vi "Tell Self Forward.vi"(6 "Msg":refnum<class "Msg.lvclass">, 7 "Actor in":refnum<class "Actor.lvclass">, 9 "Msg Attributes":T1 {"Teller"."Absolute Time" format="%<%x %.3X>T"}, 10 "Previous Told":bool) -> (0 "Error out":errorcluster, 1 "Told":bool, 2 "Told Or Previous Told":bool, 5 "Actor out":refnum<class "Actor.lvclass">)   [LabVIEW 2020, in "_Template.lvlib" / "Templates.lvlib" / "TEMPLATE jettl Msg.lvlib" / "TEMPLATE.lvlib"]
uses:
  TEMPLATE/TEMPLATE.lvlib
  jettl/jettl/jettl.lvlib
  jettl/jettl/Actor/Actor.lvclass
  jettl/jettl/Msg Input/Msg Input.lvclass
  jettl/jettl/Msg Output/Msg Output.lvclass
  jettl/jettl/Msg/Msg.lvclass
  jettl/jettl/Relation.ctl
  jettl/jettl/Teller.ctl
  jettl/jettl/Msg Attributes.ctl
panel:
  # "This front panel should not be manipulated."
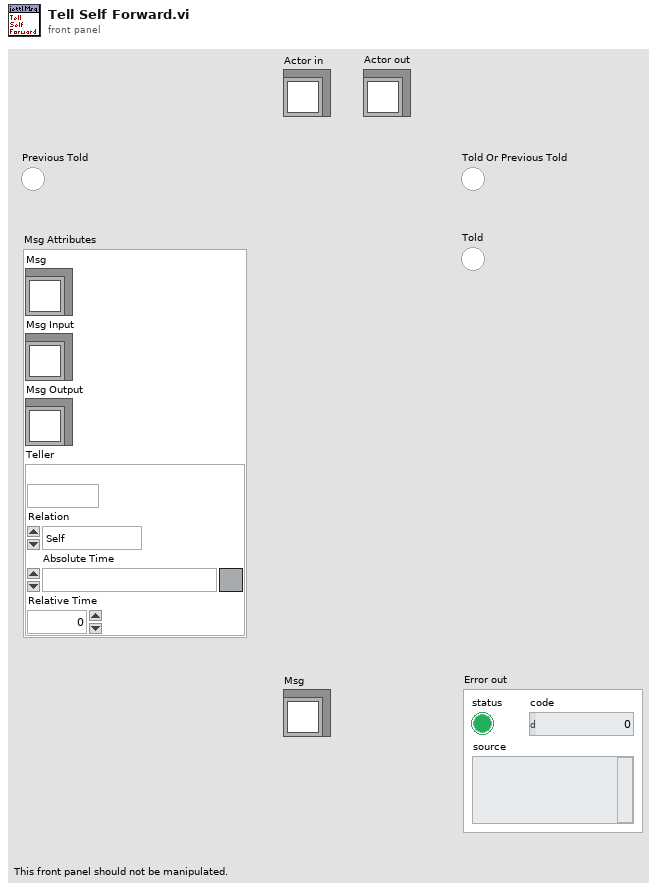
[diagram p1: front panel]
types:
  T1 = typedef "jettl.lvlib/Msg Attributes.ctl" = cluster{"Msg":refnum<class "Msg.lvclass">, "Msg Input":refnum<class "Msg Input.lvclass">, "Msg Output":refnum<class "Msg Output.lvclass">, "Teller":T2}
  T2 = typedef "jettl.lvlib/Teller.ctl" = cluster{"Alias":string, "Relation":T3, "Absolute Time":timestamp, "Relative Time":dbl}
  T3 = typedef "jettl.lvlib/Relation.ctl" = enum16{"Self", "Parent", "Child"}
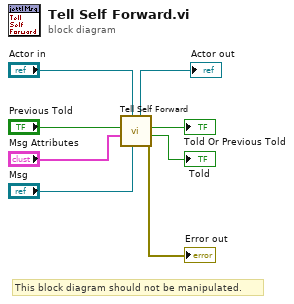
[diagram p0: block diagram]
diagram:
  # "This block diagram should not be manipulated."
  n1 = call "Tell Self Forward.vi"("Msg"="Msg", "Actor in"="Actor in", "Msg Attributes"="Msg Attributes", "Previous Told"="Previous Told") -> ("Error out"=→"Error out":errorcluster, "Told"=→"Told":bool, "Told Or Previous Told"=→"Told Or Previous Told":bool, "Actor out"=→"Actor out":refnum<class "Actor.lvclass">)  [unwired: 4 in]
